vi "Delete Menu Items.vi"(8 "error in (no error)":errorcluster, 9 "items":string, 10 "menu tag":string, 11 "Menu in":refnum<class "Menu.lvclass">) -> (0 "error out":errorcluster, 3 "Menu out":refnum<class "Menu.lvclass">)   [LabVIEW 2021, in "Menu.lvlib" / "Menu.lvclass"]
uses:
  Menu.lvclass
  Menu.lvclass/Menu.ctl
  MenuItems.ctl
  Picture2D/src/Picture/Image.lvclass
  <vilib>/Utility/miscctls.llb/LVMenuShortCut.ctl
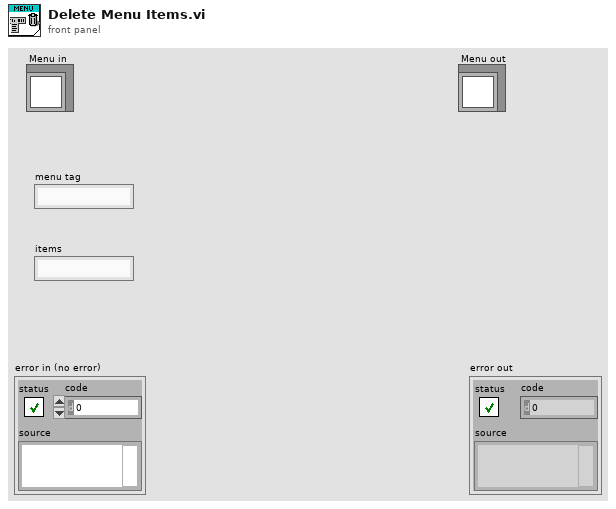
[diagram p1: front panel]
types:
  T1 = typedef "Menu.lvlib/Menu.lvclass/MenuItems.ctl" = cluster{"Item Name":string, "Short Cut":T2, "Checked":bool, "Enable":bool, "After item":string, "Item Tags":string[], "Item Names":string[], "Picture":refnum<class "Image.lvclass">, "Hilite Picture":refnum<class "Image.lvclass">, "Displayed":bool}
  T2 = typedef "LVMenuShortCut.ctl" = cluster{"Include Shift Key?":bool, "Include Ctrl Key?":bool, "Shortcut Key":string}
  T3 = typedef "Menu.lvlib/Menu.lvclass/Data.ctl" = cluster{"MenuMap":map{string, T1}, "PictRef":refnum<vi>, "MenuSelectionEvent":refnum<user-event>, "TopMenuSpacing":i32, "MenuSpacing":i32, "CloseEvent":refnum<user-event>, "TR_ManageMenuRef":refnum<vi>, "MenuColors":T4, "RTMPath":path, "RTMVIReference":refnum<vi>, "RTMMenuReference":refnum<k9>, "CtlRef":refnum<vi>, "User-Specified Font":refnum<class "Font.lvclass">, "Desired Font":enum16{"User-specified Font", "Application Font", "System Font", "Dialog Font"}, "SubMenuIcon":T5, "SubMenuIconClosed":refnum<class "Picture2D.lvclass">, "SubMenuIconOpened":refnum<class "Picture2D.lvclass">}
  T4 = typedef "Menu.lvlib/Menu.lvclass/MenuColors.ctl" = cluster{"Text":refnum<class "Color.lvclass">, "HiliteText":refnum<class "Color.lvclass">, "Background":refnum<class "Color.lvclass">, "BorderColor":refnum<class "Color.lvclass">, "Hilite":refnum<class "Color.lvclass">}
  T5 = typedef "Menu.lvlib/Menu.lvclass/SubMenuIcon.ctl" = enum16{"LabVIEW", "Windows", "Custom"}
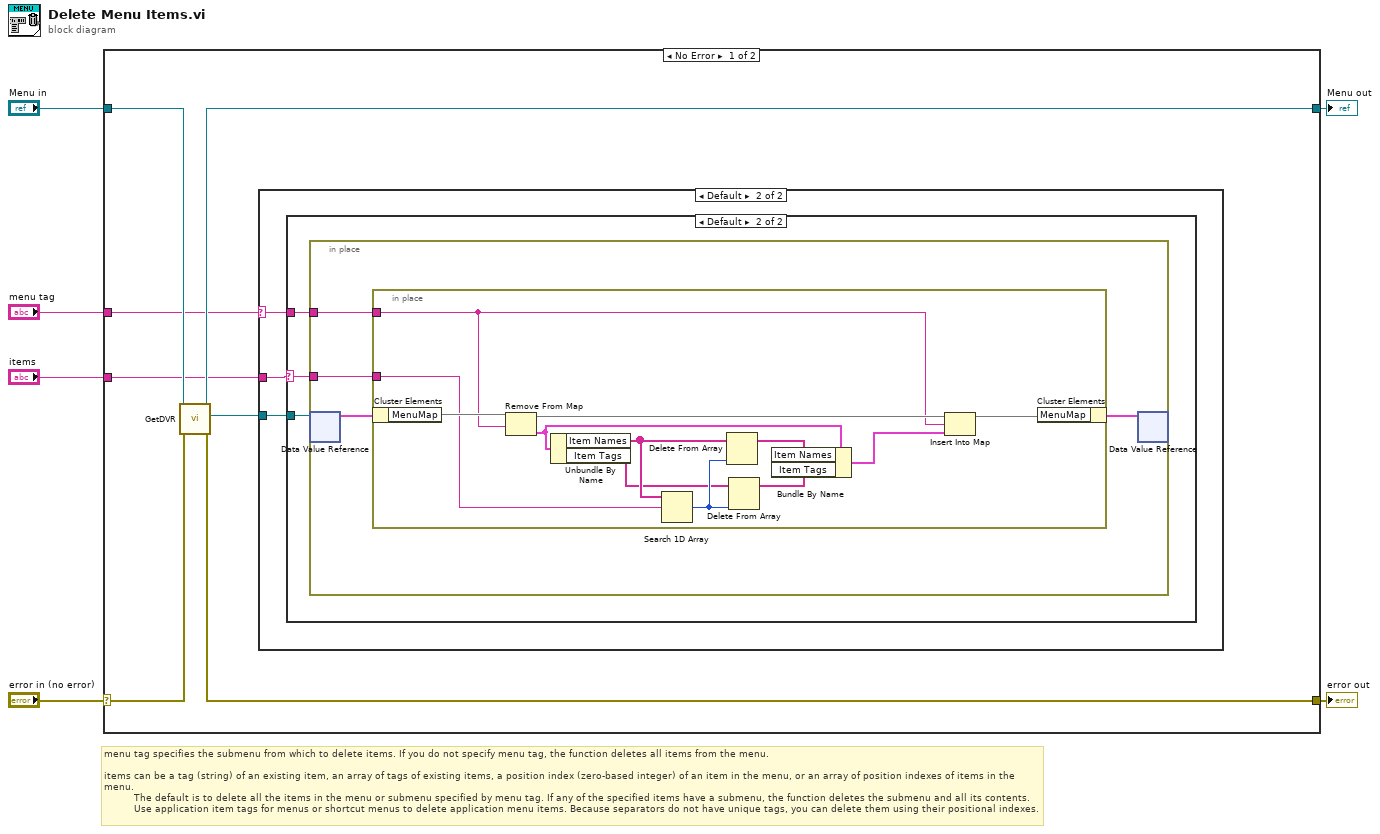
[diagram p0: block diagram]
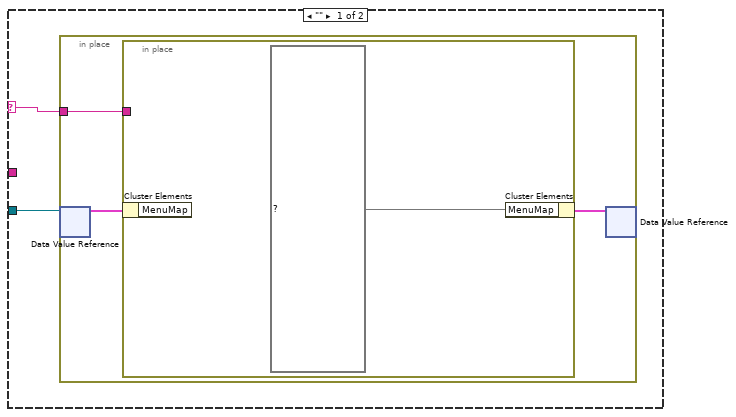
[diagram p2: hidden frame]
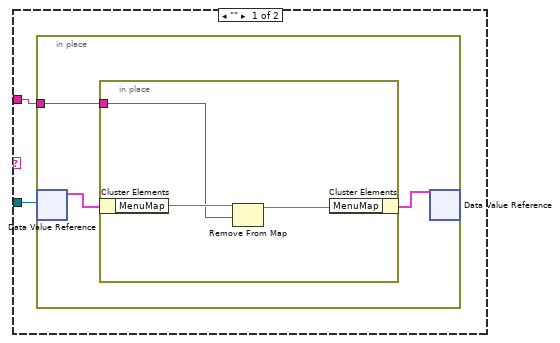
[diagram p3: hidden frame]
diagram:
  # "menu tag specifies the submenu from which to delete items. If you do not specify menu tag, the function deletes all items from the menu.  \n\nitems can be a tag (string) of an existing item, an array of tags of existing items, a position index (zero-based integer) of an item in the menu, or an array of position indexes of items in the menu. \n          The default is to delete all the items in the menu or submenu specified by menu tag. If any of the specified items have a submenu, the function deletes the submenu and all its contents. \n          Use application item tags for menus or shortcut menus to delete application menu items. Because separators do not have unique tags, you can delete them using their positional indexes."
  n1 = case shown="No Error" "error in (no error)" {
    selector: "error in (no error)" -> [w10 w51]
    tunnel: [w9 w51] -> w5
    tunnel: [w12 w50] -> w3
    tunnel: "Menu in" -> [w11 w50]
    tunnel: "menu tag" -> [w8 _]
    tunnel: "items" -> [w7 _]
    frame No Error {
      n2 = call "GetDVR.vi"("error in (no error)"=w10, "Menu in"=w11) -> ("error out"=w9:errorcluster, "DVR"=w13:refnum<data-value>, "Menu out"=w12:refnum<class "Menu.lvclass">)  [unwired: 7 in]
      n3 = case shown="Default" w8 {
        selector: w8 -> [w15 w21]
        tunnel: w13 -> [w14 w22]
        tunnel: w7 -> [_ w20]
        frame "" {
          n4 = in-place {
            in-place-border: w15 -> [w17]
            n5 = in-place-dvr #1(w14) -> (w18:T3)  [unwired: 1 out]
            n6 = in-place {
              in-place-border: w17 -> [_]
              n7 = in-place-cluster #2(w18) -> ()  [unwired: 1 out]
              n8 = in-place-cluster #2("MenuMap"=map{string, T1} {}) -> (w16:T3)
            }
            n9 = in-place-dvr #1(w16) -> ()  [unwired: 2 out]
          }
        }
        frame Default {
          n10 = case shown="Default" w20 {
            selector: w20 -> [_ w31]
            tunnel: w22 -> [w24 w33]
            tunnel: w21 -> [w23 w32]
            frame "" {
              n11 = in-place {
                in-place-border: w23 -> [w26]
                n12 = in-place-dvr #3(w24) -> (w27:T3)  [unwired: 1 out]
                n13 = in-place {
                  in-place-border: w26 -> [w28]
                  n14 = in-place-cluster #4(w27) -> ("MenuMap"=w30:map{string, T1})
                  n15 = Remove From Map(10:w28, 11:w30) -> (3:w29:map{string, T1})  [unwired: 2 out]
                  n16 = in-place-cluster #4("MenuMap"=w29) -> (w25:T3)
                }
                n17 = in-place-dvr #3(w25) -> ()  [unwired: 2 out]
              }
            }
            frame Default {
              n18 = in-place {
                in-place-border: w32 -> [w36]
                in-place-border: w31 -> [w34]
                n19 = in-place-dvr #5(w33) -> (w37:T3)  [unwired: 1 out]
                n20 = in-place {
                  in-place-border: w36 -> [w45]
                  in-place-border: w34 -> [w48]
                  n21 = in-place-cluster #6(w37) -> ("MenuMap"=w49:map{string, T1})
                  n22 = Remove From Map(10:w45, 11:w49) -> (1:w41:T1, 3:w47:map{string, T1})  [unwired: 1 out]
                  n23 = Unbundle By Name(w41) -> ("Item Names"=w44:string[], "Item Tags"=w42:string[])
                  n24 = Search 1D Array(1D array=w44, element=w48) -> (index of element=w43:i32)  [unwired: 1 in]
                  n25 = Delete From Array(array=w44, index=w43) -> (array with subset deleted=w40:string[])  [unwired: 1 in, 1 out]
                  n26 = Delete From Array(array=w42, index=w43) -> (array with subset deleted=w39:string[])  [unwired: 1 in, 1 out]
                  n27 = Bundle By Name(cluster=w41, "Item Names"=w40, "Item Tags"=w39) -> (w38:T1)
                  n28 = Insert Into Map(map in=w47, key=w45, value=w38) -> (map out=w46:map{string, T1})  [unwired: 2 out]
                  n29 = in-place-cluster #6("MenuMap"=w46) -> (w35:T3)
                }
                n30 = in-place-dvr #5(w35) -> ()  [unwired: 2 out]
              }
            }
          }
        }
      }
    }
    frame Error {
    }
  }
  "error out" <- w5
  "Menu out" <- w3
